vi "Hexapod2_GUI.vi"(10 "stop 2":refnum<vi>, 11 "GUI_cluster":T1={"Sub Panel"=refnum, "GUIdevice"="Bella_LP_Mode", "CtlRef"=refnum, "user event out"=refnum}) -> ()   [LabVIEW 2011]
uses:
  GUI_Template/GUI_master/tcp_new_data_event.ctl
  GUI_Template/GUI_master/tcp new data cluster.ctl
  Controls/GUI_cluster.ctl
  Controls/eventtypdef.ctl
panel:
  in  "relativemove.ypos::1":bool
  in  "relativemove.xpos::1":bool
  in  "relativemove.yneg::1":bool
  in  "relativemove.xneg::1":bool
  in  "relativemove.zpos::1":bool
  in  "relativemove.zneg::1":bool
  in  "relativemove.wpos::1":bool
  in  "relativemove.upos::1":bool
  in  "relativemove.uneg::1":bool
  in  "relativemove.vpos::1":bool
  in  "relativemove.vneg::1":bool
  in  "relativemove.wneg::1":bool
  in  "<command>::1":bool=TRUE
  in  "stepsize::1":dbl=0.02 caption="stepsize" min=0.0 max=10.0
  in  "wangle::1":dbl=0.19 caption="w" min=-5.0 max=5.0
  in  "vangle::1":dbl=0.0005 caption="v" min=-5.0 max=5.0
  in  "uangle::1":dbl=0.04 caption="u" min=-5.0 max=5.0
  in  "zpos::1":dbl=1.013 caption="z" min=-12.0 max=12.0
  in  "ypos::1":dbl=0.45 caption="y" min=-20.0 max=20.0
  in  "xpos::1":dbl=-1.0 caption="x" min=-20.0 max=20.0
  out "tcp data event":T2
  out "GUIdevice 1":string="StagingHexapodPI"
  in  "stop":bool
  # "+Z"
  # "+Y"
  # "-X"
  # "-Y"
  # "+X"
  # "-Z"
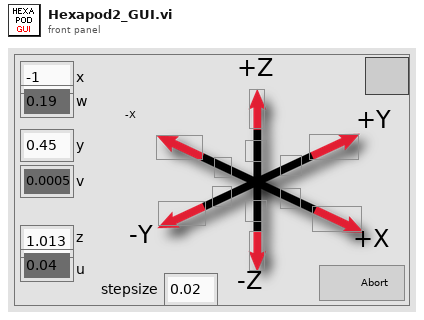
[diagram p1: front panel]
types:
  T1 = typedef "GUI_cluster.ctl" = cluster{"Sub Panel":refnum<vi>, "GUIdevice":string, "CtlRef":refnum<vi>, "user event out":refnum<user-event>}
  T2 = typedef "tcp_new_data_event.ctl" = refnum<user-event>
  T3 = typedef "eventtypdef.ctl" = cluster{"label":string, "Sub Panel":refnum<vi>, "CtlRef":refnum<vi>, "This VI":refnum<vi>}
  T4 = typedef "tcp new data cluster.ctl" = cluster{"EventEnum":enum16{"new data", "connection status update"}, "Device name":string}
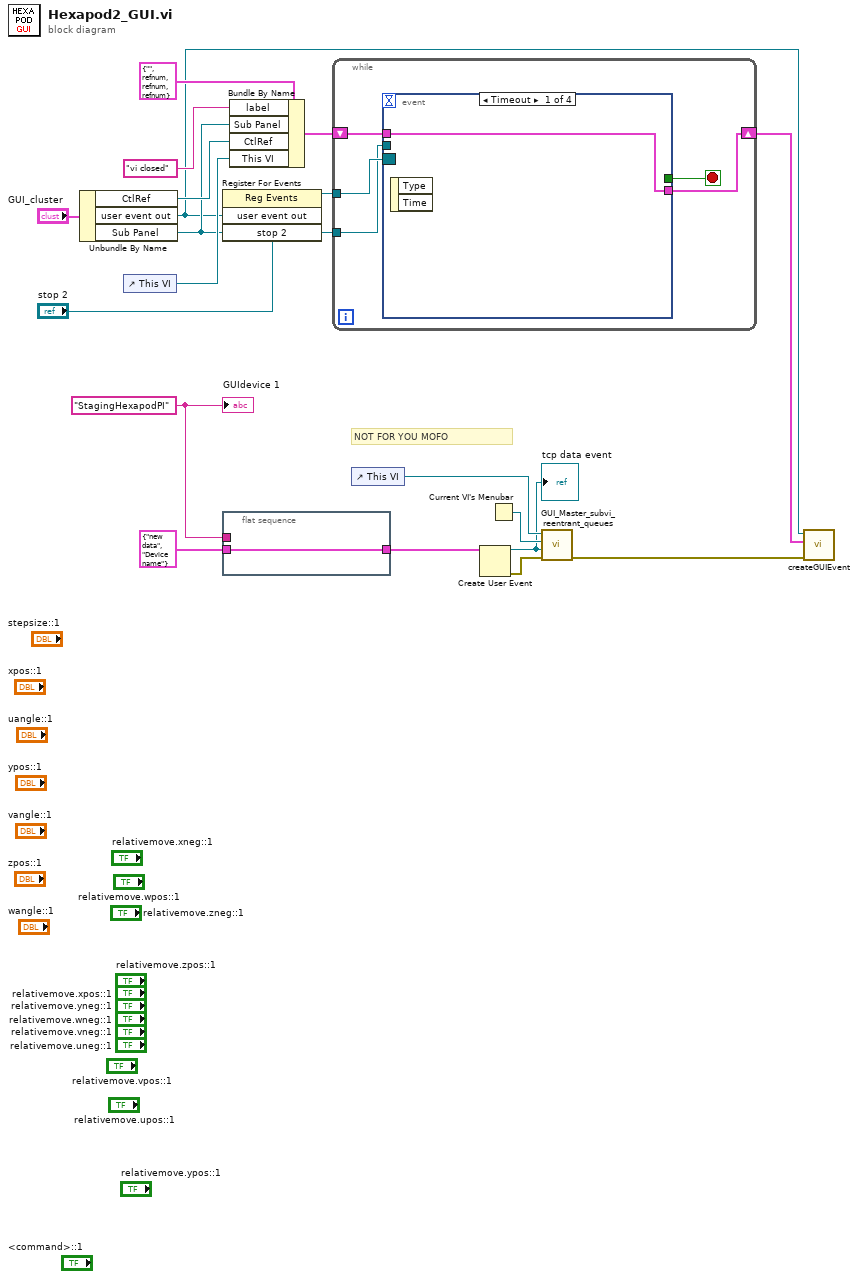
[diagram p0: block diagram]
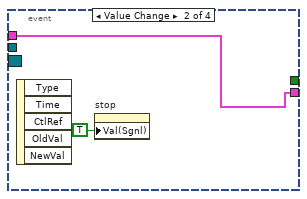
[diagram p2: hidden frame]
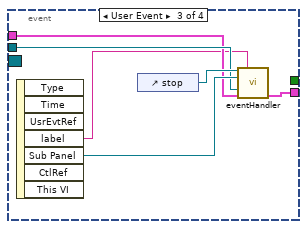
[diagram p3: hidden frame]
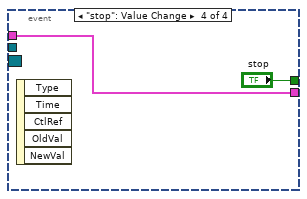
[diagram p4: hidden frame]
diagram:
  w9 = "StagingHexapodPI" ("GUIdevice")
  # "NOT FOR YOU MOFO"
  n1 = Unbundle By Name("GUI_cluster") -> ("CtlRef"=w11:refnum<vi>, "user event out"=w4:refnum<user-event>, "Sub Panel"=w6:refnum<vi>)
  n2 = control-ref of="This VI"() -> (w10:refnum<vi>)
  n3 = register-events(w4, "stop 2") -> (reference out=w8:refnum<event-registration>)  [unwired: 2 in, 1 out]
  n4 = flat-sequence {
    tunnel: T4 {"EventEnum"=enum."new data", "Device name"="Device name"} ("New Event") -> [w20]
    tunnel: [w20] -> w12
    tunnel: w9 -> [_]
    frame #0 {
    }
  }
  n5 = Bundle By Name(cluster=T3 {"label"="", "Sub Panel"=refnum, "CtlRef"=refnum, "This VI"=refnum} ("event data"), "label"="vi closed", "Sub Panel"=w6, "CtlRef"=w11, "This VI"=w10) -> (w5:T3)
  n6 = while {
    tunnel: w8 -> [w25]
    tunnel: w6 -> [w23]
    shift-right: [w21] -> w2
    shift-left: w5 -> [w22]
    stop <- w24 stop-if-true
    n7 = event shown="[0] Timeout" {
      selector: w25 -> [_ _ _ _]
      dyn-events: _ -> [_ _ _ _]
      timeout: _ -> [_ _ _ _]
      tunnel: [_ _ _ "stop"] -> w24
      tunnel: w23 -> [_ _ w32 _]
      tunnel: w22 -> [w26 w28 w31 w35]
      tunnel: [w26 w28 w30 w35] -> w21
      event Timeout {
        n8 = event-data() -> ()  [unwired: 1 in, 2 out]
      }
      event Value Change {
        n9 = event-data() -> ()  [unwired: 1 in, 5 out]
        n10 = property on="stop" class="Bool (strict)"("Val(Sgnl)"=TRUE ("Value (Signaling)")) -> ()  [unwired: 2 in, 2 out]
      }
      event User Event {
        n11 = event-data() -> ("label"=w29:string, "Sub Panel"=w33:refnum<vi>)  [unwired: 1 in, 5 out]
        n12 = control-ref of="stop"() -> (w34:refnum<vi>)
        n13 = call "eventHandler.vi"("Boolean in"=w34, "label"=w29, "Sub Panel 2"=w33, "Sub Panel"=w32, "event data in"=w31) -> ("event data out"=w30:T3)  [unwired: 10 in]
      }
      event "stop": Value Change {
        n14 = event-data() -> ()  [unwired: 1 in, 5 out]
      }
    }
  }
  n15 = control-ref of="This VI"() -> (w19:refnum<vi>)
  n16 = Create User Event(user event datatype=w12) -> (user event=w16:refnum<user-event>, error out=w17:errorcluster)  [unwired: 1 in]
  "tcp data event" <- w16
  n17 = Current VI's Menubar() -> (w18:refnum<k9>)
  n18 = call "GUI_Master_subvi_reentrant_queues.vi"("error in (no error)"=w17, "tcp data event"=w16, "Caller menu reference"=w18, "Caller VI ref"=w19) -> ("error out"=w3:errorcluster)  [unwired: 7 in]
  n19 = call "createGUIEvent.vi"("error in (no error)"=w3, "event data"=w2, "User Event in"=w4) -> ()  [unwired: 9 in]
  "GUIdevice 1" <- w9
